vi "Read State.vi"(8 "error in (no error)":errorcluster, 10 "Trigger":bool, 11 "Shutter in":refnum<class "Shutter.lvclass">) -> (0 "error out":errorcluster, 2 "Set":T1, 3 "Shutter out":refnum<class "Shutter.lvclass">)   [LabVIEW 2016, in "Shutter.lvclass"]
uses:
  Shutter.lvclass
  Controls/Shutter States.ctl
  Shutter.lvclass/Shutter.ctl
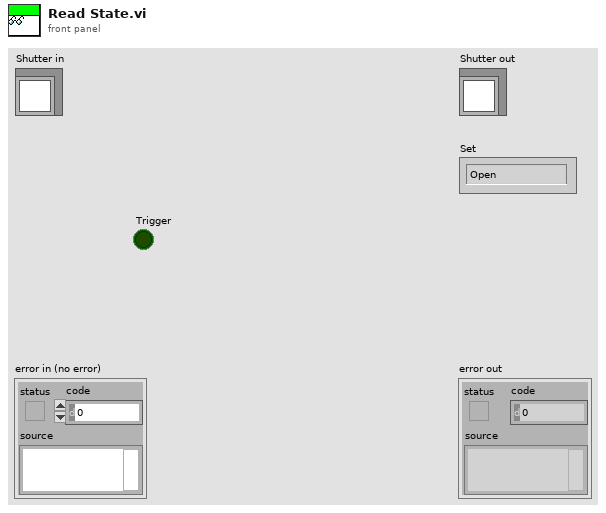
[diagram p1: front panel]
types:
  T1 = typedef "Shutter States.ctl" = enum16{"Open", "Close", "Wait", "Off", "Arm", "Idle"}
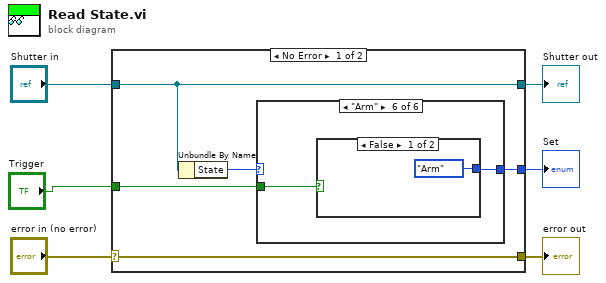
[diagram p0: block diagram]
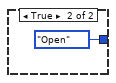
[diagram p7: hidden frame]
diagram:
  n1 = case shown="No Error" "error in (no error)" {
    selector: "error in (no error)" -> [w11 w21]
    tunnel: [w11 w21] -> w5
    tunnel: [w10 w22] -> w3
    tunnel: "Shutter in" -> [w10 w22]
    tunnel: [w8 _] -> w2
    tunnel: "Trigger" -> [w7 _]
    frame No Error {
      n2 = Unbundle By Name(w10) -> ("State"=w9:T1)
      n3 = case shown="\"Arm\"" w9 {
        selector: w9 -> [w12 w13 w14 w15 w16 _]
        tunnel: w7 -> [_ _ _ _ _ w18]
        tunnel: [w12 w13 w14 w15 w16 w17] -> w8
        frame "Open", Default {
        }
        frame "Close" {
        }
        frame "Wait" {
        }
        frame "Off" {
        }
        frame "Idle" {
        }
        frame "Arm" {
          n4 = case shown="False" w18 {
            tunnel: [Shutter_States."Arm" ("State") Shutter_States."Open" ("State")] -> w17
            frame False {
            }
            frame True {
            }
          }
        }
      }
    }
    frame Error {
    }
  }
  "error out" <- w5
  "Shutter out" <- w3
  "Set" <- w2
